vi "Framework_Initialize.vi"(8 "error in (no error)":errorcluster, 11 "AB_RESTfulWebService in":refnum<class "AB_RESTfulWebService.lvclass">) -> (0 "error out":errorcluster, 1 "helpTopics":string[](array[string]), 2 "pageTitles":string[](array[string]), 3 "AB_RESTfulWebService out":refnum<class "AB_RESTfulWebService.lvclass">, 4 "helpFile":string, 5 "pages":path[](array[path]))   [LabVIEW 2020, in "AB_RESTfulWebService.lvclass"]
uses:
  <vilib>/AppBuilder/AB_Classes/RESTful/AB_RESTfulWebService.lvclass
panel:
  in  "pageTitles_WebService":string[](array[string])=["Information", "Source Files", "URL Mappings", "Service Settings", "Destinations", "Source File Settings", "Advanced", "Additional Exclusions", "Pre/Post Build Actions", "Preview"]
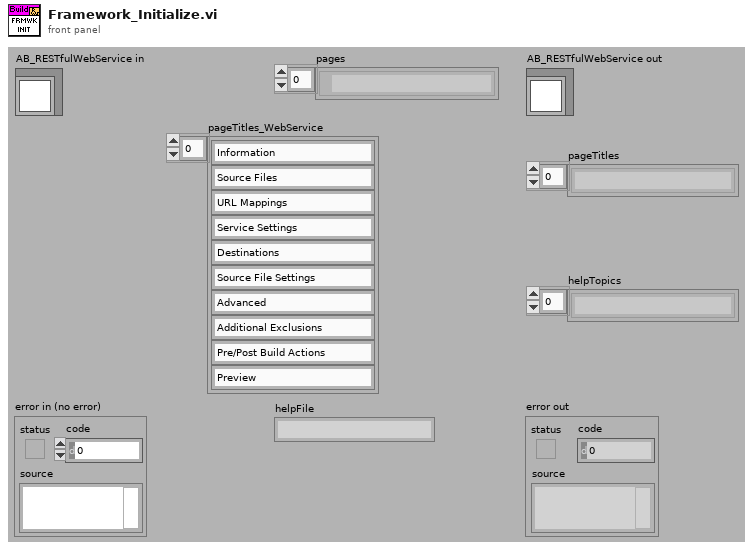
[diagram p1: front panel]
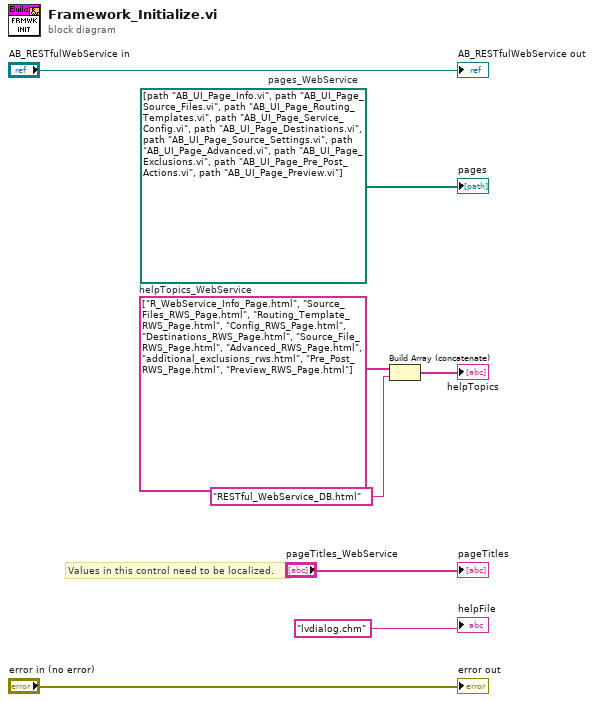
[diagram p0: block diagram]
diagram:
  w5 = string[] ["R_WebService_Info_Page.html", "Source_Files_RWS_Page.html", "Routing_Template_RWS_Page.html", "Config_RWS_Page.html", "Destinations_RWS_Page.html", "Source_File_RWS_Page.html", "Advanced_RWS_Page.html", "additional_exclusions_rws.html", "Pre_Post_RWS_Page.html", "Preview_RWS_Page.html"]  # helpTopics_WebService
  w2 = path[] [path "AB_UI_Page_Info.vi", path "AB_UI_Page_Source_Files.vi", path "AB_UI_Page_Routing_Templates.vi", path "AB_UI_Page_Service_Config.vi", path "AB_UI_Page_Destinations.vi", path "AB_UI_Page_Source_Settings.vi", path "AB_UI_Page_Advanced.vi", path "AB_UI_Page_Exclusions.vi", path "AB_UI_Page_Pre_Post_Actions.vi", path "AB_UI_Page_Preview.vi"]  # pages_WebService
  # "Values in this control need to be localized."
  n1 = Build Array (concatenate)(w5, "RESTful_WebService_DB.html" ("HTML filename")) -> (→"helpTopics":string[])
  "error out" <- "error in (no error)"
  "AB_RESTfulWebService out" <- "AB_RESTfulWebService in"
  "pages" <- w2
  "pageTitles" <- "pageTitles_WebService"
  "helpFile" <- "lvdialog.chm" ("CHM or HLP filename (lvdialog.chm)")
